vi "TLS 300.vi"() -> ()   [LabVIEW 2017, in "GUI.lvlib"]
uses:
  Libraries/GUI/GUI.lvlib
panel:
  out "Słup":T1
  out "Rezerwa":T2
  out "Pojemność KT":T3
  out "Pojemność":T4
  in  "TLS Cluster":T5
  in  "stop":bool
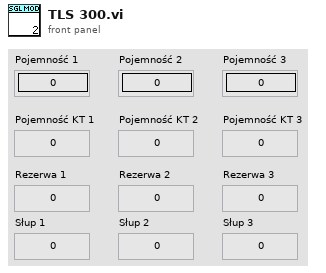
[diagram p1: front panel]
types:
  T1 = cluster{"Słup 1":dbl, "Słup 2":dbl, "Słup 3":dbl}
  T2 = cluster{"Rezerwa 1":dbl, "Rezerwa 2":dbl, "Rezerwa 3":dbl}
  T3 = cluster{"Pojemność KT 1":dbl, "Pojemność KT 2":dbl, "Pojemność KT 3":dbl}
  T4 = cluster{"Pojemność 1":dbl, "Pojemność 2":dbl, "Pojemność 3":dbl}
  T5 = cluster{"Poj":sgl[], "Poj kt":sgl[], "Rezerwa":sgl[], "Slup":sgl[]}
  T6 = cluster{"Poj[0]":sgl, "Poj[1]":sgl, "Poj[2]":sgl}
  T7 = cluster{"Poj kt[0]":sgl, "Poj kt[1]":sgl, "Poj kt[2]":sgl}
  T8 = cluster{"Rezerwa[0]":sgl, "Rezerwa[1]":sgl, "Rezerwa[2]":sgl}
  T9 = cluster{"Slup[0]":sgl, "Slup[1]":sgl, "Slup[2]":sgl}
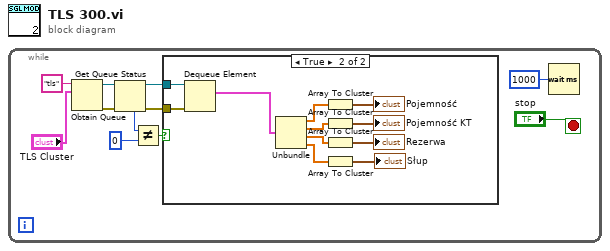
[diagram p0: block diagram]
diagram:
  n1 = while {
    stop <- "stop" stop-if-true
    n2 = Obtain Queue(name (unnamed)="tls", element data type="TLS Cluster") -> (queue out=w9:refnum<queue>, error out=w8:errorcluster)  [unwired: 3 in, 1 out]
    n3 = Get Queue Status(queue=w9, error in (no error)=w8) -> (queue out=w1:refnum<queue>, error out=w2:errorcluster, # elements in queue=w5:i32)  [unwired: 1 in, 5 out]
    n4 = Not Equal?(x=w5, y=0) -> (x != y?=w3:bool)
    n5 = case shown="True" w3 {
      tunnel: w2 -> [_ w21]
      tunnel: w1 -> [_ w22]
      frame False {
      }
      frame True {
        n6 = Dequeue Element(queue=w22, error in (no error)=w21) -> (element=w20:T5)  [unwired: 1 in, 3 out]
        n7 = Unbundle(w20) -> ("Poj"=w16:sgl[], "Poj kt"=w17:sgl[], "Rezerwa"=w18:sgl[], "Slup"=w19:sgl[])
        n8 = Array To Cluster(array=w16) -> (cluster=→"Pojemność":T6)
        n9 = Array To Cluster(array=w17) -> (cluster=→"Pojemność KT":T7)
        n10 = Array To Cluster(array=w18) -> (cluster=→"Rezerwa":T8)
        n11 = Array To Cluster(array=w19) -> (cluster=→"Słup":T9)
      }
    }
    n12 = Wait (ms)(milliseconds to wait=u32 1000) -> ()  [unwired: 1 out]
  }
